vi "ziExample-Module-PIDAdvisor.vi"() -> ()   [LabVIEW 2009]
doc: "Control a Zurich instrument device via the LabOne Labview API. \nRequirements: Zurich Instruments HF2 or UHFLI \nThis example suggests a PID configuration and sets it for an internal PLL DUT.\n\n© Zurich Instruments AG, www.zhinst.com"
uses:
  <instrlib>/Zurich Instruments LabOne/Public/ziTypeHandle.ctl
  <instrlib>/Zurich Instruments LabOne/Public/Modules/ziModSetValueBinary.vi
  <instrlib>/Zurich Instruments LabOne/Public/Configure/ziSetValueDouble.vi
  <instrlib>/Zurich Instruments LabOne/Public/Configure/ziSetValueDoubleArray.vi
  <instrlib>/Zurich Instruments LabOne/Public/Modules/ziModSetValueDouble.vi
  <instrlib>/Zurich Instruments LabOne/Public/Modules/ziModSetValueDoubleArray.vi
  <instrlib>/Zurich Instruments LabOne/Public/Modules/ziModGetDoubleData.vi
  <instrlib>/Zurich Instruments LabOne/Public/Modules/ziModGetAdvisorData.vi
  <instrlib>/Zurich Instruments LabOne/Zurich Instruments LabOne.lvlib
panel:
  out "Data":cluster{"double":dbl}[][](array[cluster])
  out "Error Out":errorcluster
  out "Handle Out":T1 {"Handle" format="0x%08x"; "Conn" format="0x%08x"}
  in  "Calculate":bool
  in  "Reset PID":bool
  out "PID OUT":dbl(graph)
  in  "stop":bool
  out "PID SHIFT":dbl(graph)
  out "PID ERROR":dbl(graph)
  in  "Address":string="DEV"
  in  "bw":dbl=1000.0 caption="target BW (Hz)"
  in  "Mode":dbl(ring)=3.0 items=["P"=1.0, "I"=2.0, "PI"=3.0, "PID"=7.0, "PIDF"=15.0]
  out "Finished?":bool
  out "i":dbl caption="I"
  out "p":dbl caption="P"
  out "dlimittimeconstant":dbl
  out "rate":dbl caption="Rate (Hz)"
  out "d":dbl caption="D"
  out "Step Response":cluster{"grid":dbl[], "r_avg":dbl[]}(graph)
  out "Bode Gain":cluster{"grid":dbl[], "r_avg":dbl[]}(graph)
  out "Bode Phase":cluster{"grid":dbl[], "r_avg":dbl[]}(graph)
  out "Selected Device":string
  in  "subscribepath":string="pidAdvisor/*" caption="Subscribe Path"
  in  "moduleID":u16(ring)=5 items=["sweep", "zoomFFT", "deviceSettings", "record", "pllAdvisor", "pidAdvisor"]
  # "ziExample-SweepModul.vi\nRequirements: UHFLI, HF2, MD/MF Option\nsee block diagram for VI description"
  # "Tested Devices:\n- UHFLI+MF \n- HF2+MF"
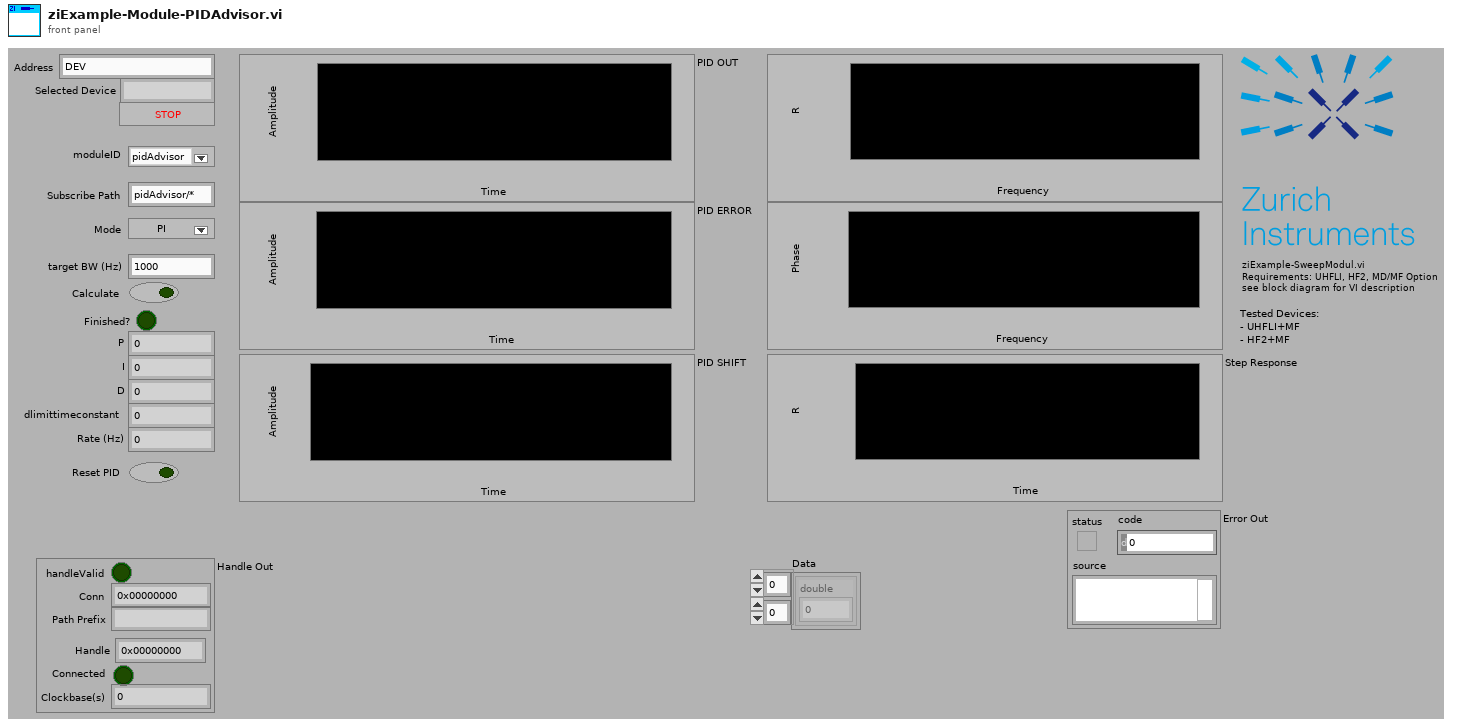
[diagram p1: front panel]
types:
  T1 = typedef "Zurich Instruments LabOne.lvlib/ziTypeHandle.ctl" = cluster{"handleValid":bool, "Conn":u64, "Path Prefix":string, "Handle":u64, "Connected":bool, "Clockbase(s)":dbl}
  T2 = typedef "Zurich Instruments LabOne.lvlib/ziTypeModHandle.ctl" = cluster{"handleValid":bool, "Conn":u64, "ModHandle":u64, "moduleID":string, "Path Prefix":string}
  T3 = typedef "Zurich Instruments LabOne.lvlib/ziTypeModResults.ctl" = cluster{"PathArray":string[], "ValueType":T4, "NoOfResults":u64, "HeaderType":enum16{"HEADER_TYPE_NONE", "HEADER_TYPE_SWTRIGGER", "HEADER_TYPE_SWEEPER"}, "ziSWTriggerHeader":T5[], "ziSweeperHeader":T6[]}
  T4 = typedef "Zurich Instruments LabOne.lvlib/ziTypePollType.ctl" = enum16{"NONE", "DOUBLE_DATA", "INTEGER_DATA", "DEMOD_SAMPLE", "SCOPE_WAVE_HF2", "AUXIN_SAMPLE", "DIO_SAMPLE", "BYTE_ARRAY", "PWA_WAVE", "9", "10", "11", "12", "13", "14", "15", "TREE_CHANGE_DEPRI", "17", "ERROR", "19", "20", "21", "22", "23", "24", "25", "26", "27", "28", "29", "30", "31", "DOUBLE_DATA_TS", "INTEGER_DATA_TS", "34", "SCOPE_WAVE", "36", "37", "BYTE_ARRAY_TS", "39", "40", "41", "42", "43", "44", "45", "CNT_DATA", "47", "TREE_CHANGE", "49", "50", "51", "52", "53", "54", "55", "56", "57", "58", "59", "60", "61", "62", "63", "SWEEPER_DATA", "SPECTRUM_DATA", "ADVISOR_DATA", "67", "IMP_DATA"}
  T5 = typedef "Zurich Instruments LabOne.lvlib/ziTypeModSWTriggerHeader.ctl" = cluster{"HeaderType":enum8{"HEADER_TYPE_NONE", "HEADER_TYPE_SWTRIGGER", "HEADER_TYPE_SWEEPER"}, "triggerStart":u64, "triggerNumber":u64, "cols":u32, "rows":u32}
  T6 = typedef "Zurich Instruments LabOne.lvlib/ziTypeModSweeperHeader.ctl" = cluster{"HeaderType":enum8{"HEADER_TYPE_NONE", "HEADER_TYPE_SWTRIGGER", "HEADER_TYPE_SWEEPER"}, "sampleFormat":u8}
  T7 = typedef "Zurich Instruments LabOne.lvlib/ziTypeModAdvisorWave.ctl" = cluster{"timestamp":u64, "sampleCount":u64, "flags":u8, "sampleFormat":u8, "grid":dbl[], "x":dbl[], "y":dbl[]}
  T8 = typedef "Zurich Instruments LabOne.lvlib/ziTypePollData.ctl" = cluster{"double":dbl, "Demod Sample":T9, "string":string, "Raw":u8[], "int":i32, "ScopeData":cluster{"wave":i16[], "dt (s)":dbl}, "DioInput":cluster{"Timestamp (ticks)":u64[], "Value":u32[]}, "AuxInput":cluster{"Timestamp (ticks)":u64[], "Val Ch0 (V)":dbl[], "Val Ch1 (V)":dbl[]}}
  T9 = typedef "Zurich Instruments LabOne.lvlib/ziTypeDemodSample.ctl" = cluster{"Channel":i32, "Timestamps (ticks)":u64[], "X (Vrms)":dbl[], "Y (Vrms)":dbl[], "Osc Phase (deg)":dbl[], "Freq (Hz)":dbl[], "DIO":u32[], "Aux In 0 (V)":dbl[], "Aux In 1 (V)":dbl[]}
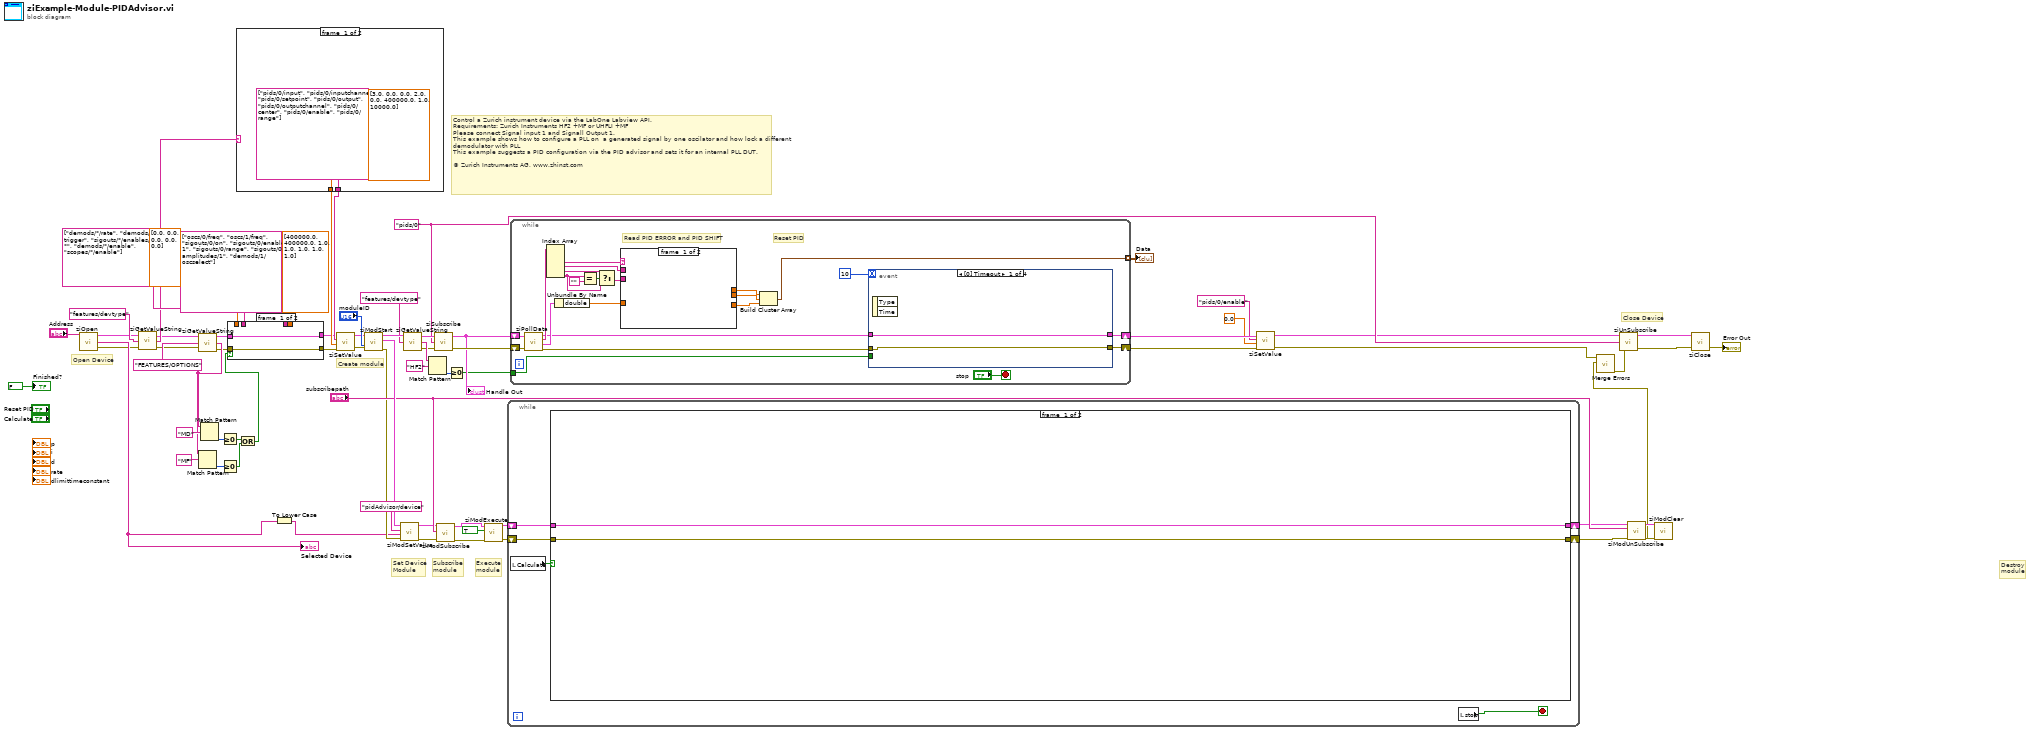
[diagram p0: block diagram]
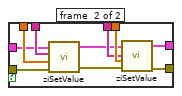
[diagram p2: hidden frame]
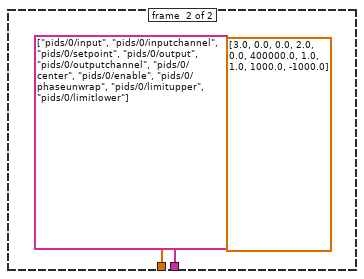
[diagram p3: hidden frame]
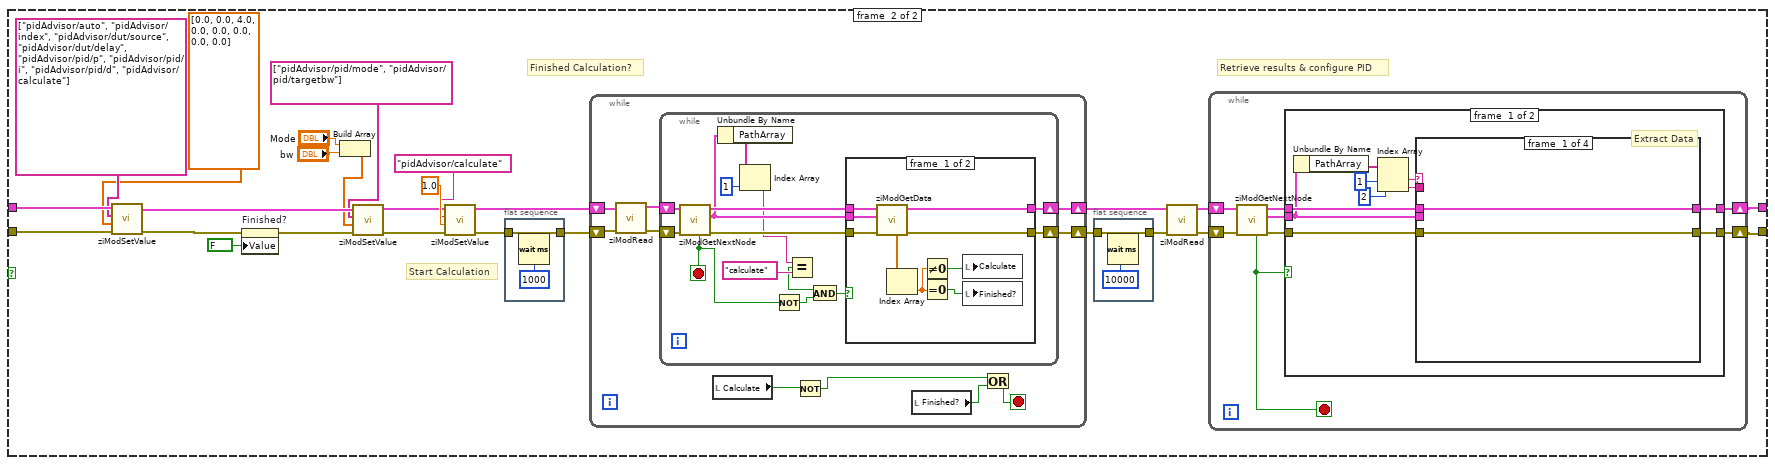
[diagram p4: hidden frame]
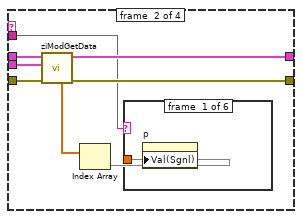
[diagram p5: hidden frame]
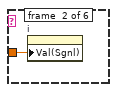
[diagram p6: hidden frame]
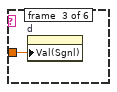
[diagram p7: hidden frame]
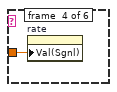
[diagram p8: hidden frame]
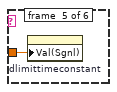
[diagram p9: hidden frame]
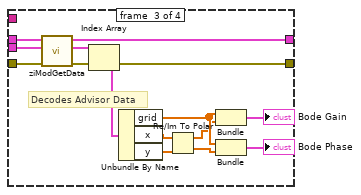
[diagram p11: hidden frame]
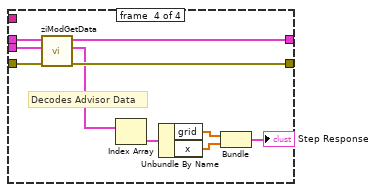
[diagram p12: hidden frame]
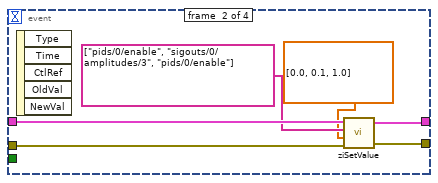
[diagram p15: hidden frame]
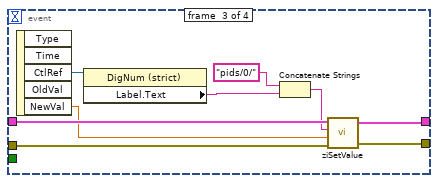
[diagram p16: hidden frame]
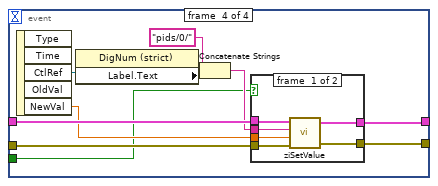
[diagram p17: hidden frame]
diagram:
  w34 = "pids/0" ("Path ()")
  # "Control a Zurich instrument device via the LabOne Labview API. \nRequirements: Zurich Instruments HF2 +MF or UHFLI +MF \nPlease connect Signal input 1 and Signall Output 1.\nThis example shows how to configure a PLL on  a generated signal by one oscilator and how lock a different demodulator with PLL\nThis example suggests a PID configuration via the PID advisor and sets it for an internal PLL DUT.\n\n© Zurich Instruments AG, www.zhinst.com"
  # "Execute\nmodule"
  # "Set Device\nModule"
  # "Subscribe\nmodule"
  # "Destroy\nmodule"
  # "Create module"
  # "Close Device"
  # "Open Device"
  n1 = call <instrlib>:"ziOpen.vi"("Address"="Address") -> ("Error Out"=w23:errorcluster, "Selected Device"=w32:string, "HandleOut"=w24:T1)  [unwired: 1 in, 2 out]
  "Selected Device" <- w32
  n2 = call <instrlib>:"ziGetValueString.vi"("error in"=w23, "Path"="features/devtype", "Handle In"=w24) -> ("error out"=w5:errorcluster, "Value"=w20:string, "Handle Out"=w4:T1)
  n3 = call <instrlib>:"ziGetValueString.vi"("error in"=w5, "Path"="FEATURES/OPTIONS", "Handle In"=w4) -> ("error out"=w2:errorcluster, "Value"=w10:string, "Handle Out"=w3:T1)
  n4 = Match Pattern(string=w10, regular expression="MF") -> (offset past match=w8:i32)  [unwired: 1 in, 3 out]
  n5 = Match Pattern(string=w10, regular expression="MD") -> (offset past match=w11:i32)  [unwired: 1 in, 3 out]
  n6 = Greater Or Equal To 0?(x=w11) -> (x >= 0?=w7:bool)
  n7 = Greater Or Equal To 0?(x=w8) -> (x >= 0?=w6:bool)
  n8 = case shown="Default" w20 {
    tunnel: [dbl[] [3.0, 0.0, 0.0, 2.0, 0.0, 400000.0, 1.0, 10000.0] dbl[] [3.0, 0.0, 0.0, 2.0, 0.0, 400000.0, 1.0, 1.0, 1000.0, -1000.0]] -> w40
    tunnel: [string[] ["pids/0/input", "pids/0/inputchannel", "pids/0/setpoint", "pids/0/output", "pids/0/outputchannel", "pids/0/center", "pids/0/enable", "pids/0/range"] string[] ["pids/0/input", "pids/0/inputchannel", "pids/0/setpoint", "pids/0/output", "pids/0/outputchannel", "pids/0/center", "pids/0/enable", "pids/0/phaseunwrap", "pids/0/limitupper", "pids/0/limitlower"]] -> w39
    frame #0 {
    }
    frame #1 {
    }
  }
  n9 = Or(x=w7, y=w6) -> (x .or. y?=w1:bool)
  n10 = case shown="True" w1 {
    tunnel: dbl[] [400000.0, 400000.0, 1.0, 1.0, 1.0, 1.0, 1.0] -> [_ w86]
    tunnel: string[] ["oscs/0/freq", "oscs/1/freq", "sigouts/0/on", "sigouts/0/enables/1", "sigouts/0/range", "sigouts/0/amplitudes/1", "demods/1/oscselect"] -> [_ w85]
    tunnel: string[] ["demods/*/rate", "demods/*/trigger", "sigouts/*/enables/*", "demods/*/enable", "scopes/*/enable"] -> [_ w82]
    tunnel: dbl[] [0.0, 0.0, 0.0, 0.0, 0.0] -> [_ w81]
    tunnel: [w76 w80] -> w22
    tunnel: [w75 w79] -> w21
    tunnel: w3 -> [w76 w78]
    tunnel: w2 -> [w75 w77]
    frame #0 {
    }
    frame #1 {
      n11 = call-poly <instrlib>:"ziSetValue.vi"("Error In"=w77, "Values"=w81, "Paths"=w82, "Handle In"=w78) -> ("Error Out"=w83:errorcluster, "Handle Out"=w84:T1)  [unwired: 1 in]
      n12 = call-poly <instrlib>:"ziSetValue.vi"("Error In"=w83, "Values"=w86, "Paths"=w85, "Handle In"=w84) -> ("Error Out"=w79:errorcluster, "Handle Out"=w80:T1)  [unwired: 1 in]
    }
  }
  n13 = To Lower Case(string=w32) -> (all lower case string=w31:string)
  n14 = call-poly <instrlib>:"ziSetValue.vi"("Error In"=w21, "Values"=w40, "Paths"=w39, "Handle In"=w22) -> ("Error Out"=w68:errorcluster, "Handle Out"=w69:T1)  [unwired: 1 in]
  n15 = call <instrlib>:"ziModStart.vi"("Error In"=w68, "module Id"="moduleID", "Handle In"=w69) -> ("Error Out"=w44:errorcluster, "ModHandle Out"=w65:T2, "Handle Out"=w51:T1)  [unwired: 6 in]
  n16 = call-poly <instrlib>:"ziModSetValue.vi"("Error In"=w44, "Data"=w31, "Path"="pidAdvisor/device", "ModHandle In"=w65) -> ("Error Out"=w55:errorcluster, "ModHandle Out"=w54:T2)  [unwired: 6 in]
  n17 = call <instrlib>:"ziGetValueString.vi"("Path"="features/devtype", "Handle In"=w51) -> ("error out"=w43:errorcluster, "Value"=w48:string, "Handle Out"=w50:T1)  [unwired: 1 in]
  n18 = Match Pattern(string=w48, regular expression="HF2") -> (offset past match=w47:i32)  [unwired: 1 in, 3 out]
  n19 = call <instrlib>:"ziSubscribe.vi"("error in"=w43, "Path ()"=w34, "Handle In"=w50) -> ("error out"=w66:errorcluster, "Handle Out"=w52:T1)  [unwired: 1 in]
  "Handle Out" <- w52
  n20 = call <instrlib>:"ziModSubscribe.vi"("Error In"=w55, "Path"="subscribepath", "ModHandle In"=w54) -> ("Error Out"=w62:errorcluster, "ModHandle Out"=w61:T2)  [unwired: 6 in]
  n21 = Greater Or Equal To 0?(x=w47) -> (x >= 0?=w46:bool)
  n22 = call <instrlib>:"ziModExecute.vi"("Error In"=w62, "Modal (F)"=TRUE ("Modal"), "ziModHandle In"=w61) -> ("Error Out"=w63:errorcluster, "ziModHandle Out"=w53:T2)  [unwired: 5 in, 1 out]
  n23 = while {
    shift-right: [w90] -> w15
    shift-left: w53 -> [w89]
    shift-right: [w91] -> w14
    shift-left: w63 -> [w88]
    stop <- w92 stop-if-true
    n24 = local read "Calculate"() -> (w87:bool)
    n25 = case shown="True" w87 {
      tunnel: w89 -> [w93 w112]
      tunnel: w88 -> [w94 w113]
      tunnel: [w94 w95] -> w91
      tunnel: [w93 w96] -> w90
      frame #0 {
      }
      frame #1 {
        # "Extract Data"
        # "Retrieve results & configure PID"
        # "Finished Calculation?"
        # "Start Calculation"
        n26 = call-poly <instrlib>:"ziModSetValue.vi"("Error In"=w113, "Values"=dbl[] [0.0, 0.0, 4.0, 0.0, 0.0, 0.0, 0.0, 0.0], "Paths"=string[] ["pidAdvisor/auto", "pidAdvisor/index", "pidAdvisor/dut/source", "pidAdvisor/dut/delay", "pidAdvisor/pid/p", "pidAdvisor/pid/i", "pidAdvisor/pid/d", "pidAdvisor/calculate"], "ModHandle In"=w112) -> ("Error Out"=w99:errorcluster, "ModHandle Out"=w105:T2)  [unwired: 6 in]
        n27 = property on="Finished?" class="Bool (strict)"(error in=w99, "Value"=FALSE ("Finished?")) -> (error out=w100:errorcluster)  [unwired: 1 in, 1 out]
        n28 = Build Array("Mode", "bw") -> (w102:dbl[])
        n29 = call-poly <instrlib>:"ziModSetValue.vi"("Error In"=w100, "Values"=w102, "Paths"=string[] ["pidAdvisor/pid/mode", "pidAdvisor/pid/targetbw"], "ModHandle In"=w105) -> ("Error Out"=w101:errorcluster, "ModHandle Out"=w111:T2)  [unwired: 6 in]
        n30 = call-poly <instrlib>:"ziModSetValue.vi"("Error In"=w101, "Value"=1.0, "Path"="pidAdvisor/calculate", "ModHandle In"=w111) -> ("Error Out"=w110:errorcluster, "ModHandle Out"=w118:T2)  [unwired: 6 in]
        n31 = flat-sequence {
          tunnel: [w124] -> w109
          tunnel: w110 -> [w124]
          frame #0 {
            n32 = Wait (ms)(milliseconds to wait=u32 1000) -> ()  [unwired: 1 out]
          }
        }
        n33 = while {
          shift-right: [w193] -> w119
          shift-left: w118 -> [w191]
          shift-right: [w192] -> w98
          shift-left: w109 -> [w190]
          stop <- w186 stop-if-true
          n34 = call <instrlib>:"ziModRead.vi"("error in"=w190, "ziModHandle In"=w191) -> ("error out"=w189:errorcluster, "ziModHandle Out"=w188:T2)  [unwired: 8 in]
          n35 = while {
            shift-right: [w203] -> w193
            shift-left: w188 -> [w207]
            shift-right: [w202] -> w192
            shift-left: w189 -> [w208]
            stop <- w195 stop-if-true
            n36 = call <instrlib>:"ziModGetNextNode.vi"("Error In"=w208, "ModHandle In"=w207) -> ("Error Out"=w205:errorcluster, "ModResults"=w204:T3, "ModHandle Out"=w206:T2, "NoData"=w195:bool)  [unwired: 6 in]
            n37 = Unbundle By Name(w204) -> ("PathArray"=w201:string[])
            n38 = Index Array(array=w201, index=1) -> (element=w199:string)
            n39 = Not(x=w195) -> (.not. x?=w194:bool)
            n40 = Equal?(x=w199, y="calculate") -> (x = y?=w196:bool)
            n41 = And(x=w196, y=w194) -> (x .and. y?=w197:bool)
            n42 = case shown="False" w197 {
              tunnel: w206 -> [w217 w219]
              tunnel: w204 -> [w216 _]
              tunnel: w205 -> [w215 w218]
              tunnel: [w214 w218] -> w202
              tunnel: [w213 w219] -> w203
              frame #0 {
                n43 = call-poly <instrlib>:"ziModGetData.vi"("Error In"=w215, "ModResults"=w216, "ModHandle In"=w217) -> ("Error Out"=w214:errorcluster, "ModHandle Out"=w213:T2, "Value"=w211:dbl[])  [unwired: 4 in, 2 out]
                n44 = Index Array(array=w211) -> (element=w210:dbl)  [unwired: 1 in]
                n45 = Not Equal To 0?(x=w210) -> (x != 0?=w209:bool)
                n46 = Equal To 0?(x=w210) -> (x = 0?=w212:bool)
                n47 = local write "Calculate"(w209) -> ()
                n48 = local write "Finished?"(w212) -> ()
              }
              frame #1 {
              }
            }
          }
          n49 = local read "Calculate"() -> (w185:bool)
          n50 = Not(x=w185) -> (.not. x?=w184:bool)
          n51 = local read "Finished?"() -> (w187:bool)
          n52 = Or(x=w184, y=w187) -> (x .or. y?=w186:bool)
        }
        n53 = flat-sequence {
          tunnel: w98 -> [w121]
          tunnel: [w121] -> w97
          frame #0 {
            n54 = Wait (ms)(milliseconds to wait=u32 10000) -> ()  [unwired: 1 out]
          }
        }
        n55 = call <instrlib>:"ziModRead.vi"("error in"=w97, "ziModHandle In"=w119) -> ("error out"=w115:errorcluster, "ziModHandle Out"=w116:T2)  [unwired: 8 in]
        n56 = while {
          shift-right: [w126] -> w96
          shift-left: w116 -> [w131]
          shift-right: [w125] -> w95
          shift-left: w115 -> [w132]
          stop <- w127 stop-if-true
          n57 = call <instrlib>:"ziModGetNextNode.vi"("Error In"=w132, "ModHandle In"=w131) -> ("Error Out"=w129:errorcluster, "ModResults"=w128:T3, "ModHandle Out"=w130:T2, "NoData"=w127:bool)  [unwired: 6 in]
          n58 = case shown="False" w127 {
            tunnel: w130 -> [w142 w183]
            tunnel: w129 -> [w141 w182]
            tunnel: w128 -> [w136 _]
            tunnel: [w140 w183] -> w126
            tunnel: [w139 w182] -> w125
            frame #0 {
              n59 = Unbundle By Name(w136) -> ("PathArray"=w134:string[])
              n60 = Index Array(array=w134, index #1=1 ("index"), index #2=2 ("index")) -> (element #1=w138:string, element #2=w135:string)
              n61 = case shown="\"pid\"" w138 {
                tunnel: w142 -> [w144 w152 w170 w180]
                tunnel: w136 -> [_ w151 w171 w181]
                tunnel: w141 -> [w143 w150 w169 w179]
                tunnel: [w143 w147 w168 w178] -> w139
                tunnel: [w144 w149 w167 w177] -> w140
                tunnel: w135 -> [_ w146 _ _]
                frame #0 {
                }
                frame #1 {
                  n62 = call-poly <instrlib>:"ziModGetData.vi"("Error In"=w150, "ModResults"=w151, "ModHandle In"=w152) -> ("Error Out"=w147:errorcluster, "ModHandle Out"=w149:T2, "Value"=w145:dbl[])  [unwired: 4 in, 2 out]
                  n63 = Index Array(array=w145) -> (element=w148:dbl)  [unwired: 1 in]
                  n64 = case shown="\"rate\"" w146 {
                    tunnel: w148 -> [w153 w154 w155 w156 w157 _]
                    frame #0 {
                      n65 = property on="p" class="DigNum (strict)"("Val(Sgnl)"=w153) -> ()  [unwired: 2 in, 2 out]
                    }
                    frame #1 {
                      n66 = property on="i" class="DigNum (strict)"("Val(Sgnl)"=w154) -> ()  [unwired: 2 in, 2 out]
                    }
                    frame #2 {
                      n67 = property on="d" class="DigNum (strict)"("Val(Sgnl)"=w155) -> ()  [unwired: 2 in, 2 out]
                    }
                    frame #3 {
                      n68 = property on="rate" class="DigNum (strict)"("Val(Sgnl)"=w156) -> ()  [unwired: 2 in, 2 out]
                    }
                    frame #4 {
                      n69 = property on="dlimittimeconstant" class="DigNum (strict)"("Val(Sgnl)"=w157) -> ()  [unwired: 2 in, 2 out]
                    }
                    frame #5 {
                    }
                  }
                }
                frame #2 {
                  # "Decodes Advisor Data"
                  n70 = call-poly <instrlib>:"ziModGetData.vi"("Error In"=w169, "ModResults"=w171, "ModHandle In"=w170) -> ("Error Out"=w168:errorcluster, "AdvisorData Out"=w165:T7[], "ModHandle Out"=w167:T2)  [unwired: 6 in]
                  n71 = Index Array(array=w165) -> (element=w166:T7)  [unwired: 1 in]
                  n72 = Unbundle By Name(w166) -> ("grid"=w162:dbl[], "x"=w158:dbl[], "y"=w159:dbl[])
                  n73 = Re/Im To Polar(2:w159, 3:w158) -> (0:w160:dbl[], 1:w161:dbl[])
                  n74 = Bundle("grid"=w162, w161) -> (→"Bode Gain":cluster{"grid":dbl[], dbl[]})  [unwired: 1 in]
                  n75 = Bundle("grid"=w162, w160) -> (→"Bode Phase":cluster{"grid":dbl[], dbl[]})  [unwired: 1 in]
                }
                frame #3 {
                  # "Decodes Advisor Data"
                  n76 = call-poly <instrlib>:"ziModGetData.vi"("Error In"=w179, "ModResults"=w181, "ModHandle In"=w180) -> ("Error Out"=w178:errorcluster, "AdvisorData Out"=w175:T7[], "ModHandle Out"=w177:T2)  [unwired: 6 in]
                  n77 = Index Array(array=w175) -> (element=w176:T7)  [unwired: 1 in]
                  n78 = Unbundle By Name(w176) -> ("grid"=w174:dbl[], "x"=w173:dbl[])
                  n79 = Bundle("grid"=w174, "x"=w173) -> (→"Step Response":cluster{"grid":dbl[], "x":dbl[]})  [unwired: 1 in]
                }
              }
            }
            frame #1 {
              (unwired) FALSE
            }
          }
        }
      }
    }
    n80 = local read "stop"() -> (w92:bool)
  }
  n81 = while {
    shift-right: [w230] -> w29
    shift-left: w52 -> [w236]
    shift-right: [w231] -> w30
    shift-left: w66 -> [w235]
    tunnel: w46 -> [w224]
    tunnel: [w220] -> w37 mode=indexing
    stop <- "stop" stop-if-true
    # "Reset PID"
    # "Read PID ERROR and PID SHIFT"
    n82 = call <instrlib>:"ziPollData.vi"("Error In"=w235, "Handle In"=w236) -> ("Error Out"=w232:errorcluster, "Data Out"=w240:T8, "PathArray"=w239:string[], "Handle Out"=w233:T1)  [unwired: 4 in, 2 out]
    n83 = Index Array(array=w239) -> (element #2=w242:string, element #3=w241:string, element #4=w227:string, element #5=w226:string)  [unwired: 5 in, 1 out]
    n84 = Unbundle By Name(w240) -> ("double"=w238:dbl)
    n85 = Equal?(x=w226, y="") -> (x = y?=w228:bool)
    n86 = Select(t=w227, s=w228, f=w226) -> (s? t:f=w225:string)
    n87 = case shown="\"PIDS\"" w242 {
      tunnel: w241 -> [_ w283]
      tunnel: w225 -> [_ w282]
      tunnel: w238 -> [_ w281]
      tunnel: [_ w280] -> w223
      tunnel: [_ w279] -> w222
      tunnel: [_ w278] -> w221
      frame #0 {
      }
      frame #1 {
        n88 = case shown="\"0\"" w283 {
          tunnel: w282 -> [_ w288]
          tunnel: w281 -> [_ w287]
          tunnel: [_ w286] -> w280
          tunnel: [_ w285] -> w279
          tunnel: [_ w284] -> w278
          frame #0 {
          }
          frame #1 {
            n89 = case shown="\"False\", Default" w288 {
              tunnel: w287 -> [_ w289 w290 w291]
              tunnel: [_ _ _ w291] -> w286
              tunnel: [_ w289 _ _] -> w285
              tunnel: [_ _ w290 _] -> w284
              frame #0 {
              }
              frame #1 {
                "PID ERROR" <- w289
              }
              frame #2 {
                "PID OUT" <- w290
              }
              frame #3 {
                "PID SHIFT" <- w291
              }
            }
          }
        }
      }
    }
    n90 = Build Cluster Array(w221, w222, w223) -> (w220:cluster{"double":dbl}[])
    n91 = event shown="[0] Timeout" {
      selector: _ -> [_ _ _ _]
      dyn-events: _ -> [_ _ _ _]
      timeout: 10 -> [_ _ _ _]
      tunnel: w233 -> [w244 w250 w259 w269]
      tunnel: [w244 w249 w258 w268] -> w230
      tunnel: w232 -> [w243 w248 w257 w267]
      tunnel: [w243 w247 w256 w266] -> w231
      tunnel: w224 -> [_ _ _ w260]
      event #0 {
        n92 = event-data() -> ()  [unwired: 1 in, 2 out]
      }
      event #1 {
        n93 = event-data() -> ()  [unwired: 1 in, 5 out]
        n94 = call-poly <instrlib>:"ziSetValue.vi"("Error In"=w248, "Values"=dbl[] [0.0, 0.1, 1.0], "Paths"=string[] ["pids/0/enable", "sigouts/0/amplitudes/3", "pids/0/enable"], "Handle In"=w250) -> ("Error Out"=w247:errorcluster, "Handle Out"=w249:T1)  [unwired: 1 in]
      }
      event #2 {
        n95 = event-data() -> ("CtlRef"=w254:refnum<vi>, "NewVal"=w255:dbl)  [unwired: 1 in, 3 out]
        n96 = property on="Property Node" class="DigNum (strict)"(reference=w254) -> ("Label.Text"=w252:string)  [unwired: 1 in, 2 out]
        n97 = Concatenate Strings("pids/0/" ("string"), w252) -> (w251:string)
        n98 = call-poly <instrlib>:"ziSetValue.vi"("Error In"=w257, "Value"=w255, "Path"=w251, "Handle In"=w259) -> ("Error Out"=w256:errorcluster, "Handle Out"=w258:T1)  [unwired: 1 in]
      }
      event #3 {
        n99 = event-data() -> ("CtlRef"=w264:refnum<vi>, "NewVal"=w265:dbl)  [unwired: 1 in, 3 out]
        n100 = property on="Property Node" class="DigNum (strict)"(reference=w264) -> ("Label.Text"=w262:string)  [unwired: 1 in, 2 out]
        n101 = Concatenate Strings("pids/0/" ("string"), w262) -> (w261:string)
        n102 = case shown="False" w260 {
          tunnel: w269 -> [w275 w277]
          tunnel: [w274 w277] -> w268
          tunnel: w267 -> [w273 w276]
          tunnel: [w272 w276] -> w266
          tunnel: w265 -> [w271 _]
          tunnel: w261 -> [w270 _]
          frame #0 {
            n103 = call-poly <instrlib>:"ziSetValue.vi"("Error In"=w273, "Value"=w271, "Path"=w270, "Handle In"=w275) -> ("Error Out"=w272:errorcluster, "Handle Out"=w274:T1)  [unwired: 1 in]
          }
          frame #1 {
          }
        }
      }
    }
  }
  "Data" <- w37
  n104 = call-poly <instrlib>:"ziSetValue.vi"("Error In"=w30, "Value"=0.0, "Path"="pids/0/enable", "Handle In"=w29) -> ("Error Out"=w18:errorcluster, "Handle Out"=w28:T1)  [unwired: 1 in]
  n105 = call <instrlib>:"ziModUnSubscribe.vi"("Error In"=w14, "Path (\"/\")"="subscribepath", "ModHandle In"=w15) -> ("Error Out"=w56:errorcluster, "ModHandle Out"=w57:T2)  [unwired: 7 in]
  n106 = call <instrlib>:"ziModClear.vi"("Error In"=w56, "ziModHandle In"=w57) -> ("Error Out"=w19:errorcluster)  [unwired: 7 in, 1 out]
  n107 = call <vilib>:"Merge Errors.vi"("error in 2 (no error)"=w19, "error in 1 (no error)"=w18) -> ("error out"=w16:errorcluster)  [unwired: 5 in]
  n108 = call <instrlib>:"ziUnSubscribe.vi"("error in"=w16, "Path (\"/\")"=w34, "Handle in"=w28) -> ("error out"=w17:errorcluster, "Handle out"=w33:T1)  [unwired: 1 in]
  n109 = call <instrlib>:"ziClose.vi"("Error In"=w17, "Handle In"=w33) -> ("Error Out"=→"Error Out":errorcluster)  [unwired: 2 in, 1 out]
  "Finished?" <- FALSE ("Finished?")
